vi "Configure Control.vi"(8 "error in":errorcluster, 11 "TEC 1090 in":refnum<class "Meerstetter TEC.lvclass">) -> (0 "error out":errorcluster, 2 "Setpoint":sgl, 3 "TEC 1090 out":refnum<class "Meerstetter TEC.lvclass">)   [LabVIEW 2014, in "Meerstetter Lib.lvlib" / "Meerstetter TEC.lvclass"]
uses:
  Meerstetter TEC.lvclass
  Meerstetter TEC.lvclass/Meerstetter TEC.ctl
  Controls/Input Selection.ctl
  Controls/Target temp source.ctl
  Controls/Sine ramp start point.ctl
  Controls/Output Selection.ctl
  Configurable Device/Configurable Device.lvclass/Configurable Device.ctl
  reusable/Session APIs/File Access/Config Data/Config Data.lvclass/Config Data.ctl
  Configurable Device/Read ID.vi
  Configurable Device/Read Handle.vi
  reusable/Session APIs/File Access/Config Data/Accessors/Read Ref.vi
  Configurable Device/Write Device Active_.vi
  Accessors/Read ctlVal.vi
  <vilib>/Utility/config.llb/Read Key (Double).vi
  <vilib>/Utility/config.llb/Read Key (String).vi
  reusable/Session APIs/File Access/Config Data/Config Data.lvclass
  <vilib>/Utility/config.llb/NI_LVConfig.lvlib
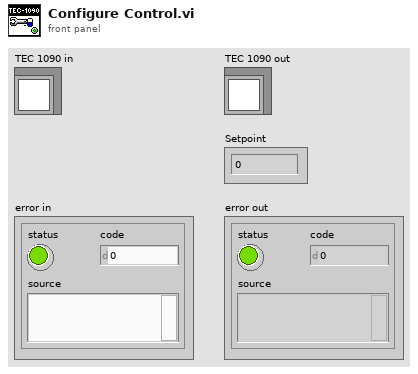
[diagram p1: front panel]
types:
  T1 = typedef "Meerstetter Lib.lvlib/Meerstetter TEC.lvclass/Ctl Method.ctl" = enum16{"Temperature", "Power"}
  T2 = typedef "Meerstetter Lib.lvlib/Meerstetter TEC.lvclass/Output Selection.ctl" = enum16{"Static OFF", "Static ON", "Live OFF/ON", "HW Enable"}
  T3 = typedef "Meerstetter Lib.lvlib/Meerstetter TEC.lvclass/Sine ramp start point.ctl" = enum16{"Measured temp", "Target temp"}
  T4 = typedef "Meerstetter Lib.lvlib/Meerstetter TEC.lvclass/Target temp source.ctl" = enum16{"Target Object Temp", "Object Target Temp"}
  T5 = typedef "Meerstetter Lib.lvlib/Meerstetter TEC.lvclass/Input Selection.ctl" = enum16{"Static Current/Voltage", "Live Current/Voltage", "Temperature Controller"}
  T6 = typedef "Config Data.lvclass/Config Session.ctl" = refnum<data-value>
  T7 = typedef "NI_LVConfig.lvlib/Config Data RefNum.ctl" = refnum<k1>
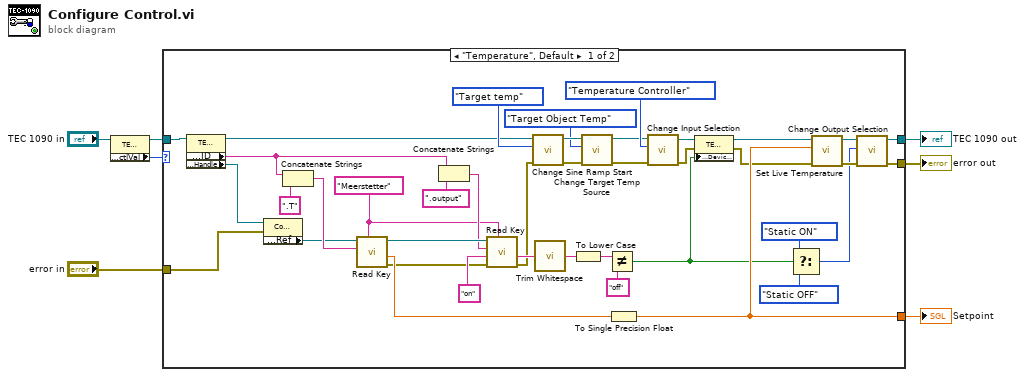
[diagram p0: block diagram]
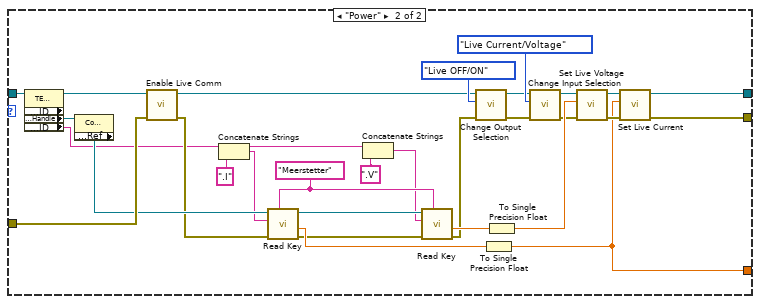
[diagram p2: hidden frame]
diagram:
  n1 = property class="TEC 1090"(reference="TEC 1090 in") -> (reference out=w1:refnum<class "Meerstetter TEC.lvclass">, "Accessors:ctlVal"=w2:T1)  [unwired: 1 in, 1 out]
  n2 = case shown="\"Temperature\", Default" w2 {
    tunnel: w1 -> [w22 w59]
    tunnel: [w37 w72] -> w5
    tunnel: [w35 w67] -> w6
    tunnel: "error in" -> [w12 w60]
    tunnel: [w45 w66] -> w4
    frame "Temperature", Default {
      w15 = "Meerstetter" ("section")
      n3 = property class="TEC 1090"(reference=w22) -> (reference out=w21:refnum<class "Meerstetter TEC.lvclass">, "Accessors:ID"=w17:string, "Accessors:Handle"=w14:T6)  [unwired: 1 in, 1 out]
      n4 = property class="Config Data"(reference=w14, error in=w12) -> ("Accessors:Ref"=w13:T7)  [unwired: 2 out]
      n5 = Concatenate Strings(w17, ".T" ("input 2")) -> (w16:string)
      n6 = call-poly <vilib>:"Read Key.vi"("section"=w15, "key"=w16, "refnum"=w13) -> ("error out"=w11:errorcluster, "value"=w46:dbl, "refnum out"=w34:T7)  [unwired: 5 in, 1 out]
      n7 = Concatenate Strings(w17, ".output" ("input 2")) -> (w19:string)
      n8 = call-poly <vilib>:"Read Key.vi"("section"=w15, "error in (no error)"=w11, "default value"="on", "key"=w19, "refnum"=w34) -> ("error out"=w10:errorcluster, "value"=w33:string)  [unwired: 3 in, 2 out]
      n9 = call "Change Sine Ramp Start.vi"("error in"=w10, "Start point"=Sine_ramp_start_point."Target temp", "TEC 1090 in"=w21) -> ("error out"=w40:errorcluster, "TEC 1090 out"=w43:refnum<class "Meerstetter TEC.lvclass">)  [unwired: 7 in]
      n10 = call <vilib>:"Trim Whitespace.vi"("string"=w33) -> ("trimmed string"=w32:string)  [unwired: 1 in]
      n11 = To Lower Case(string=w32) -> (all lower case string=w31:string)
      n12 = call "Change Target Temp Source.vi"("error in"=w40, "Target temp source"=Target_temp_source."Target Object Temp", "TEC 1090 in"=w43) -> ("error out"=w39:errorcluster, "TEC 1090 out"=w44:refnum<class "Meerstetter TEC.lvclass">)  [unwired: 7 in]
      n13 = Not Equal?(x=w31, y="off") -> (x != y?=w24:bool)
      n14 = To Single Precision Float(number=w46) -> (single precision float=w45:sgl)
      n15 = call "Change Input Selection.vi"("error in"=w39, "Input Selection"=Input_Selection."Temperature Controller", "TEC 1090 in"=w44) -> ("error out"=w9:errorcluster, "TEC 1090 out"=w26:refnum<class "Meerstetter TEC.lvclass">)  [unwired: 7 in]
      n16 = property class="TEC 1090"(reference=w26, error in=w9, "Accessors:Device Active_"=w24) -> (reference out=w25:refnum<class "Meerstetter TEC.lvclass">, error out=w8:errorcluster)
      n17 = Select(t=Output_Selection."Static ON" ("f"), s=w24, f=Output_Selection."Static OFF" ("Output Selection")) -> (s? t:f=w29:T2)
      n18 = call "Set Live Temperature.vi"("error in"=w8, "T"=w45, "TEC 1090 in"=w25) -> ("error out"=w36:errorcluster, "TEC 1090 out"=w38:refnum<class "Meerstetter TEC.lvclass">)  [unwired: 7 in]
      n19 = call "Change Output Selection.vi"("error in"=w36, "Output Selection"=w29, "TEC 1090 in"=w38) -> ("error out"=w35:errorcluster, "TEC 1090 out"=w37:refnum<class "Meerstetter TEC.lvclass">)  [unwired: 7 in]
    }
    frame "Power" {
      w58 = "Meerstetter" ("section")
      n20 = property class="TEC 1090" props=["Accessors:ID", "Accessors:Handle", "Accessors:ID"](reference=w59) -> (reference out=w57:refnum<class "Meerstetter TEC.lvclass">, "Accessors:Handle"=w56:T6, "Accessors:ID"=w50:string)  [unwired: 1 in, 2 out]
      n21 = property class="Config Data"(reference=w56) -> ("Accessors:Ref"=w55:T7)  [unwired: 1 in, 2 out]
      n22 = call "Enable Live Comm.vi"("error in"=w60, "TEC 1090 in"=w57) -> ("error out"=w52:errorcluster, "TEC 1090 out"=w61:refnum<class "Meerstetter TEC.lvclass">)  [unwired: 8 in]
      n23 = Concatenate Strings(w50, ".I" ("input 2")) -> (w53:string)
      n24 = call-poly <vilib>:"Read Key.vi"("section"=w58, "error in (no error)"=w52, "key"=w53, "refnum"=w55) -> ("error out"=w48:errorcluster, "value"=w75:dbl, "refnum out"=w77:T7)  [unwired: 4 in, 1 out]
      n25 = Concatenate Strings(w50, ".V" ("input 2")) -> (w49:string)
      n26 = call-poly <vilib>:"Read Key.vi"("section"=w58, "error in (no error)"=w48, "key"=w49, "refnum"=w77) -> ("error out"=w63:errorcluster, "value"=w76:dbl)  [unwired: 4 in, 2 out]
      n27 = call "Change Output Selection.vi"("error in"=w63, "Output Selection"=Output_Selection."Live OFF/ON", "TEC 1090 in"=w61) -> ("error out"=w62:errorcluster, "TEC 1090 out"=w65:refnum<class "Meerstetter TEC.lvclass">)  [unwired: 7 in]
      n28 = To Single Precision Float(number=w75) -> (single precision float=w66:sgl)
      n29 = To Single Precision Float(number=w76) -> (single precision float=w74:sgl)
      n30 = call "Change Input Selection.vi"("error in"=w62, "Input Selection"=Input_Selection."Live Current/Voltage", "TEC 1090 in"=w65) -> ("error out"=w69:errorcluster, "TEC 1090 out"=w71:refnum<class "Meerstetter TEC.lvclass">)  [unwired: 7 in]
      n31 = call "Set Live Voltage.vi"("error in"=w69, "V"=w74, "TEC 1090 in"=w71) -> ("error out"=w68:errorcluster, "TEC 1090 out"=w73:refnum<class "Meerstetter TEC.lvclass">)  [unwired: 7 in]
      n32 = call "Set Live Current.vi"("error in"=w68, "I"=w66, "TEC 1090 in"=w73) -> ("error out"=w67:errorcluster, "TEC 1090 out"=w72:refnum<class "Meerstetter TEC.lvclass">)  [unwired: 7 in]
    }
  }
  "error out" <- w6
  "TEC 1090 out" <- w5
  "Setpoint" <- w4
